vi "Is Door Open.vi"(0 "Interface_object in":refnum<class "Door.lvclass">, 5 "error in (no error)":errorcluster) -> (14 "Interface_object out":refnum<class "Door.lvclass">, 16 "Is Door Open?":bool, 19 "error out":errorcluster)   [LabVIEW 2018, in "Door.lvclass"]
uses:
  Door.lvclass
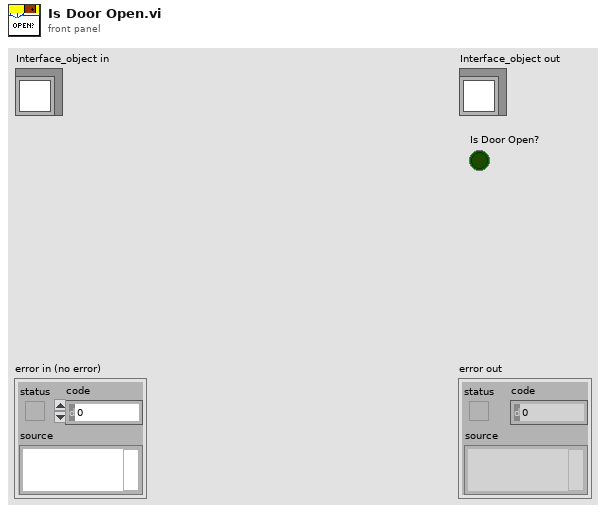
[diagram p1: front panel]
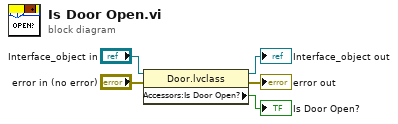
[diagram p0: block diagram]
diagram:
  n1 = property class="Door.lvclass"(reference="Interface_object in", error in="error in (no error)") -> (reference out=→"Interface_object out":refnum<class "Door.lvclass">, error out=→"error out":errorcluster, "Accessors:Is Door Open?"=→"Is Door Open?":bool)
